vi "UpdateWeightsHidden1.vi"(0 "Input":sgl[](array[numeric]), 1 "OutH1":sgl[](array[numeric])=[0.0, 0.0, 0.0, 0.0], 2 "OutH2":sgl[](array[numeric])=[0.0, 0.0, 0.0, 0.0], 3 "dEOut_dOut":sgl, 4 "Output":sgl, 5 "Learning Rate":sgl) -> ()   [LabVIEW 2020]
uses:
  <vilib>/rvi/Emulation/niFpgaSctlEmulationGetInTimedLoop.vi
  Global var FPGA.vi
  <vilib>/rvi/Memory/Memory_Emulation/nirvimemoryFastEmulation.vi
  <vilib>/rvi/Memory/Memory_Emulation/nirvimemoryEmulation.vi
  <vilib>/rvi/Emulation/niFpgaEmulationIsFPGAContextNoSignature.vi
  <vilib>/rvi/DataTransferAndStorage/Container/Common/niFpgaContainerGetUniqueNameForEmu.vi
  <vilib>/rvi/Emulation/niFpgaProcessEmulError.vi
  <vilib>/rvi/errors/nirviReportUnexpectedCaseInternalError (U32).vi
  <vilib>/rvi/DataTransferAndStorage/Container/XNode/niFpgaContainer.xnode
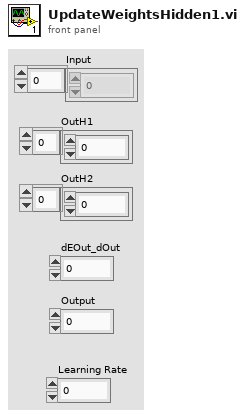
[diagram p1: front panel]
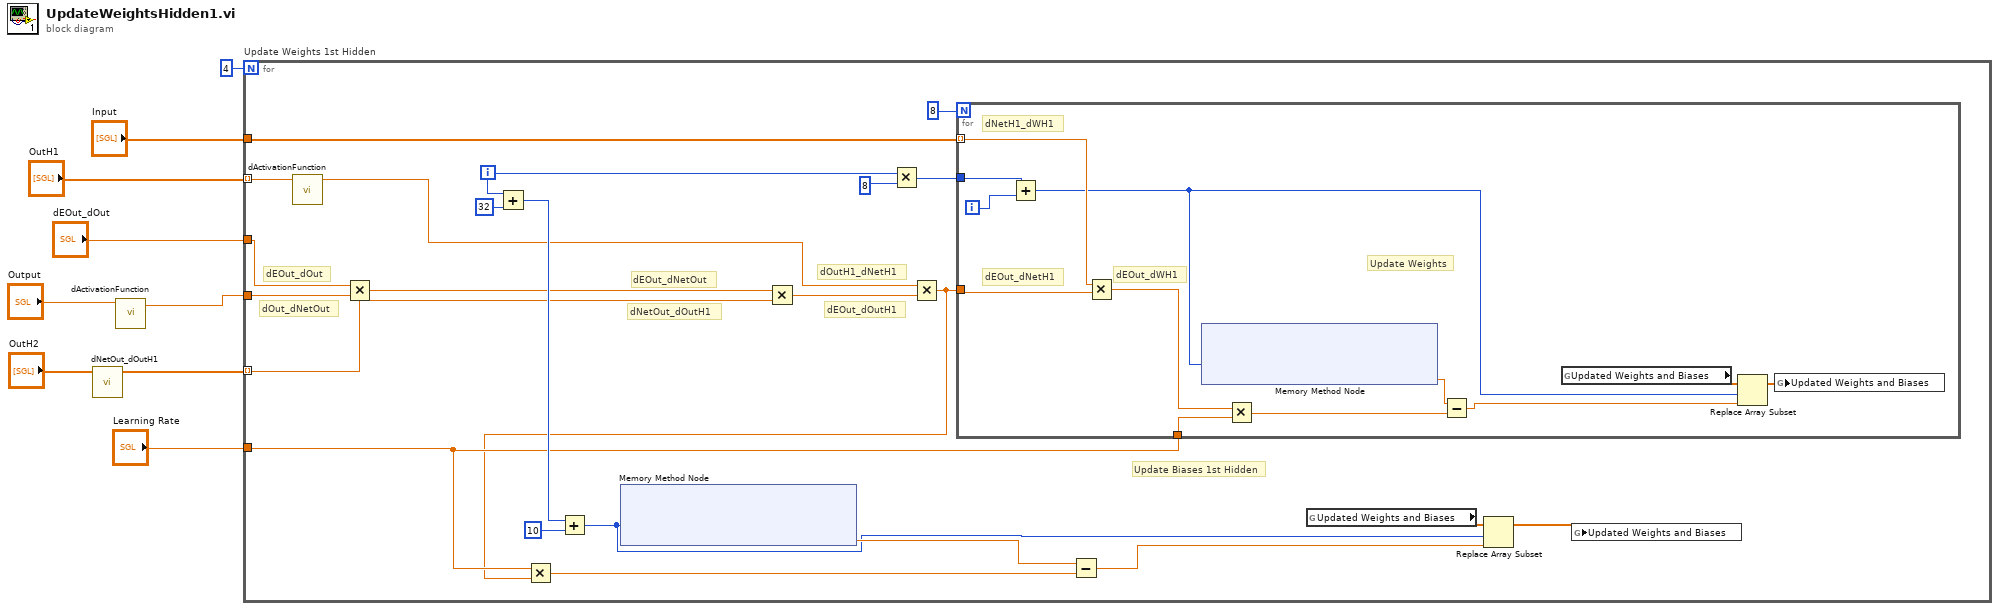
[diagram p0: block diagram]
diagram:
  n1 = call "dNetOut_dOutH1.vi"("OutH2"="OutH2") -> ("Output"=w7:sgl[])  [unwired: 10 in]
  n2 = call "dActivationFunction.vi"("Output"="Output") -> ("f"=w1:sgl)  [unwired: 10 in]
  n3 = for "Update Weights 1st Hidden" {
    N: 4 -> [_]
    tunnel: "OutH1" -> [w24] mode=indexing
    tunnel: "dEOut_dOut" -> [w15]
    tunnel: "Learning Rate" -> [w28]
    tunnel: w7 -> [w18] mode=indexing
    tunnel: "Input" -> [w17]
    tunnel: w1 -> [w16]
    i -> [w23]
    # "dOut_dNetOut"
    # "dEOut_dOut"
    # "dEOut_dOutH1"
    # "dNetOut_dOutH1"
    # "dOutH1_dNetH1"
    # "dEOut_dNetOut"
    # "Update Biases 1st Hidden"
    n4 = call "dActivationFunction.vi"("Output"=w24) -> ("f"=w20:sgl)  [unwired: 10 in]
    n5 = Multiply(x=w15, y=w16) -> (x*y=w14:sgl)
    n6 = Add(x=w23, y=32) -> (x+y=w31:i32)
    n7 = Add(x=w31, y=10) -> (x+y=w11:i32)
    n8 = xnode ("Memory Method Node")("Address"=w11) -> ("Data"=w27:sgl)  [unwired: 1 in, 1 out]
    n9 = Multiply(x=w14, y=w18) -> (x*y=w21:sgl)
    n10 = Multiply(x=w23, y=8 ("x")) -> (x*y=w26:i32)
    n11 = Multiply(x=w20, y=w21) -> (x*y=w19:sgl)
    n12 = Multiply(x=w28, y=w19) -> (x*y=w29:sgl)
    n13 = for {
      N: 8 -> [_]
      tunnel: w26 -> [w44]
      tunnel: w28 -> [w43]
      tunnel: w19 -> [w38]
      tunnel: w17 -> [w37] mode=indexing
      i -> [w39]
      # "dEOut_dNetH1"
      # "dNetH1_dWH1"
      # "dEOut_dWH1"
      # "Update Weights"
      n14 = Add(x=w44, y=w39) -> (x+y=w33:i32)
      n15 = Multiply(x=w37, y=w38) -> (x*y=w42:sgl)
      n16 = xnode ("Memory Method Node")("Address"=w33) -> ("Data"=w41:sgl)  [unwired: 1 in, 1 out]
      n17 = Multiply(x=w42, y=w43) -> (x*y=w40:sgl)
      n18 = Subtract(x=w41, y=w40) -> (x-y=w34:sgl)
      n19 = global read "Global var FPGA.vi" "Updated Weights and Biases"() -> (w36:sgl[])
      n20 = Replace Array Subset(array=w36, new element=w34, index=w33) -> (w35:sgl[])
      n21 = global write "Global var FPGA.vi" "Updated Weights and Biases"(w35) -> ()
    }
    n22 = Subtract(x=w27, y=w29) -> (x-y=w10:sgl)
    n23 = global read "Global var FPGA.vi" "Updated Weights and Biases"() -> (w13:sgl[])
    n24 = Replace Array Subset(array=w13, new element=w10, index=w11) -> (w12:sgl[])
    n25 = global write "Global var FPGA.vi" "Updated Weights and Biases"(w12) -> ()
  }
